vi "Create UserEventHandler.vi"(8 "error in":errorcluster, 9 "Level":T1, 10 "Name":string) -> (0 "error out":errorcluster, 3 "UserEventHandler out":refnum<class "UserEventHandler.lvclass">)   [LabVIEW 2024, in "hse-logger.lvlib" / "UserEventHandler.lvclass"]
doc: "Creates and initializes a new UserEventHandler object.\n\n____\nHAMPEL SOFTWARE ENGINEERING v2.2.2 (2025-01-16 15:41)"
uses:
  <vilib>/Hampel Software Engineering/HSE Logger/Handler/UserEventHandler/UserEventHandler.lvclass
  <vilib>/Hampel Software Engineering/HSE Logger/LogLevel.ctl
  <vilib>/Hampel Software Engineering/HSE Logger/hse-logger.lvlib
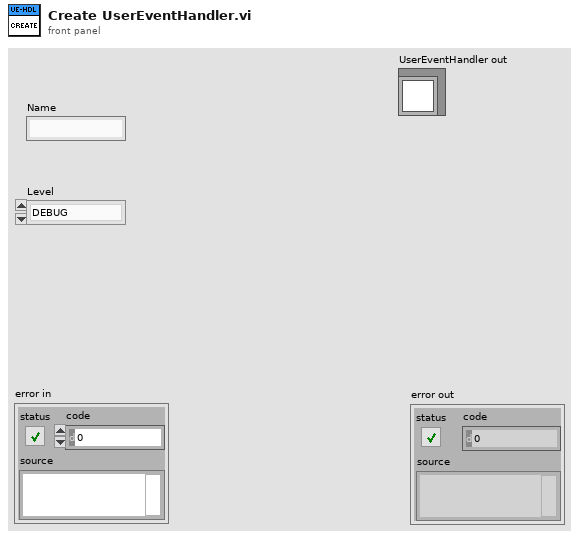
[diagram p1: front panel]
types:
  T1 = typedef "hse-logger.lvlib/LogLevel.ctl" = enum16{"DEBUG", "INFO", "WARNING", "ERROR", "CRITICAL"}
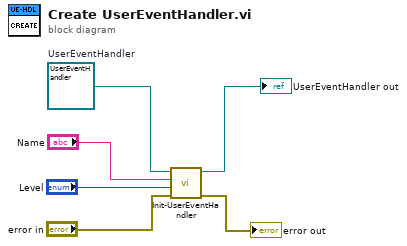
[diagram p0: block diagram]
diagram:
  w3 = refnum<class "UserEventHandler.lvclass"> refnum  # UserEventHandler
  n1 = call-dynamic "Init-UserEventHandler.vi"("error in"="error in", "Level"="Level", "Name"="Name", "UserEventHandler"=w3) -> ("error out"=→"error out":errorcluster, "UserEventHandler out"=→"UserEventHandler out":refnum<class "UserEventHandler.lvclass">)  [unwired: 6 in]
